vi "Untitled 2.vi"() -> ()   [LabVIEW 2015]
uses:
  <instrlib>/u-blox 5 Series/u-blox 5 Series.lvlib
panel:
  out "error out":errorcluster
  out "VISA resource name out":refnum<visa-resource-name>
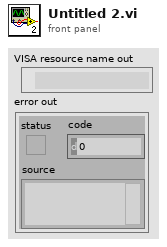
[diagram p1: front panel]
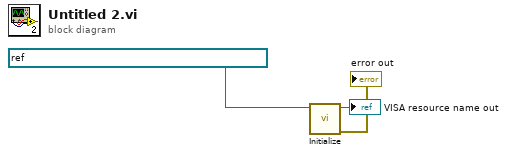
[diagram p0: block diagram]
diagram:
  n1 = call <instrlib>:"Initialize.vi"("VISA resource name"=refnum<visa-resource-name> "USB0::0x1546::0x01A8::NI-VISA-1003::1::RAW") -> ("error out"=→"error out":errorcluster, "VISA resource name out"=→"VISA resource name out":refnum<visa-resource-name>)  [unwired: 9 in]
